vi "TDS_ReadAllChannels.vi"(8 "error in":errorcluster, 11 "VI Server ClusterDUP":T1) -> (0 "error out":errorcluster)   [LabVIEW 2020]
uses:
  Instance           1 33Saved   SQUIB_TDS_ReadAllChannels .vi
  LabVIEW 2020 Toolkits/VI Server Toolkit/VI Server Libraries/VI Server_GetControl.llb/VI Server_ComboBox_Get.vi
  NA-E5071B/E5071B.llb/Labels&Control References.ctl
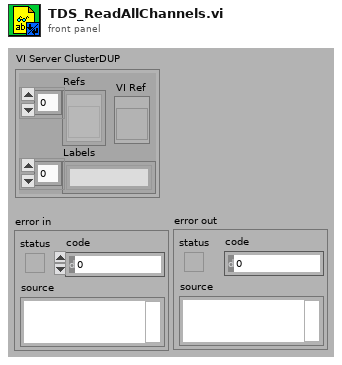
[diagram p1: front panel]
types:
  T1 = typedef "Labels&Control References.ctl" = cluster{"Refs":refnum<vi>[], "Labels":string[], "VI Ref":refnum<vi>}
  T2 = typedef "VI Server_RefsCluster.ctl" = cluster{"Labels":string[], "Refs":refnum<vi>[], "VI Ref":refnum<vi>}
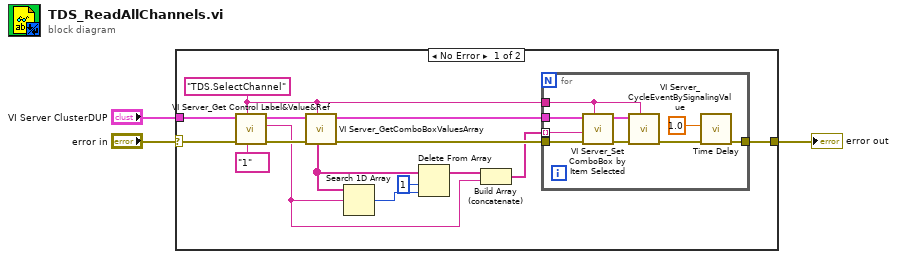
[diagram p0: block diagram]
diagram:
  n1 = case shown="No Error" "error in" {
    selector: "error in" -> [w18 w28]
    tunnel: "VI Server ClusterDUP" -> [w14 _]
    tunnel: [w7 w28] -> w2
    frame No Error {
      w8 = "TDS.SelectChannel" ("Label")
      n2 = call-poly "VI Server_Get Control Label&Value&Ref.vi"("DataType"="1" ("Default Value"), "Control.Label"=w8, "error in"=w18, "VI Server.RefsCluster"=w14) -> ("error out"=w16:errorcluster, "Value"=w4:string, "VI Server.RefsCluster.DUP"=w15:T2)  [unwired: 4 in, 1 out]
      n3 = call <userlib>:"VI Server_GetComboBoxValuesArray.vi"("Label"=w8, "error in"=w16, "Data Cluster"=w15) -> ("error out"=w10:errorcluster, "Data Cluster dup"=w9:T1, "Values[]"=w13:string[])  [unwired: 4 in, 2 out]
      n4 = Search 1D Array(1D array=w13, element=w4) -> (index of element=w12:i32)  [unwired: 1 in]
      n5 = Delete From Array(array=w13, length=1, index=w12) -> (array with subset deleted=w6:string[])  [unwired: 1 out]
      n6 = Build Array (concatenate)(w6, w4) -> (w5:string[])
      n7 = for {
        tunnel: w10 -> [w27]
        tunnel: w9 -> [w26]
        tunnel: w8 -> [w25]
        tunnel: [w19] -> w7
        tunnel: w5 -> [w23] mode=indexing
        n8 = call "VI Server_Set ComboBox by Item Selected.vi"("Label"=w25, "error in"=w27, "ComboBoxValue"=w23, "Data Cluster"=w26) -> ("error out"=w22:errorcluster, "Data Cluster dup"=w24:T1)  [unwired: 5 in, 1 out]
        n9 = call "VI Server_CycleEventBySignalingValue.vi"("Label"=w25, "error in"=w22, "VI Server Cluster"=w24) -> ("error out"=w20:errorcluster)  [unwired: 7 in, 1 out]
        n10 = call "Time Delay"("error in (no error)"=w20, "Delay Time (s)"=1.0) -> ("error out"=w19:errorcluster)  [unwired: 9 in]
      }
    }
    frame Error {
    }
  }
  "error out" <- w2
